vi "Fire Private Event.vi"(7 "AdHoc Cmd (\"\")":string, 8 "error in (no error)":errorcluster, 9 "vData":variant, 10 "PrivAsync":T1, 11 "Main in":refnum<class "Main.lvclass">) -> (0 "error out":errorcluster, 3 "Main out":refnum<class "Main.lvclass">)   [LabVIEW 2019, in "Main.lvclass"]
doc: "Developed by Kevin Thompson\nkevin@thompsonengineering.net\n\nCopyright 2018\nThompson Engineering, LLC"
uses:
  Main.lvclass
  DataTypes/PrivateAsynEv_Main--enum.ctl
  Common/DataTypes/TD Async CmdMsg EventData--cluster.ctl
  Main.lvclass/Main.ctl
  Accessors/Get ObjData.vi
  Config/Config.lvclass
  DAQ_Engine/DAQ_Engine.lvclass
  Log_Engine/Log_Engine.lvclass
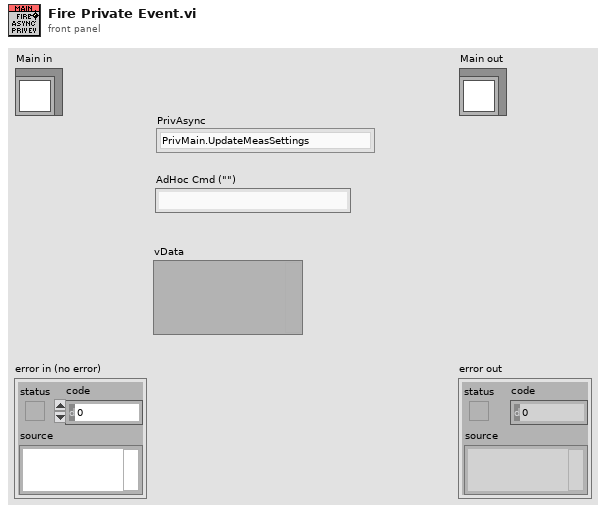
[diagram p1: front panel]
types:
  T1 = typedef "Main.lvclass/PrivateAsynEv_Main--enum.ctl" = enum16{"PrivMain.UpdateMeasSettings", "PrivMain.UpdateAcqMode", "PrivMain.UpdateDAQState", "PrivMain.UpdateLogState", "PrivMain.UpdateTDMSState", "PrivMain.UpdateProcessingState", "PrivMain.Stop&Terminate", "PrivMain.CurrInverterUpdated", "PrivMain.UpdateStoreUseESRBaseline", "PrivMain.SetUnsetAlarm&ESRBLine", "PrivMain.ResetAveraging"}
  T2 = typedef "TD Async CmdMsg EventData--cluster.ctl" = cluster{"Time Stamp":timestamp, "CmdMsg":string, "vData":variant}
  T3 = typedef "Main.lvclass/ObjData--cluster.ctl" = cluster{"Settings":T4, "Public Events":T7, "Dependency":T8, "ReadData-placeholder":T9, "VISA-placeholder":refnum<visa-resource-name>, "InverterWaveformsQ":T10, "Application.TerminateProcess Event":refnum<user-event>, "RawDaqDataQ":T11, "MeasSettings":T12, "InverterDataAcqMode":T13, "DAQState Data":T14, "Private Events":T16, "InvWfmsQ-DT":T10, "DPAuxDataQ":T17, "ProcessingState":T18, "InverterInfo":T19, "CurrInverters":T20[], "InverterLUT Dict":T24, "ESR Chart Ref":refnum<vi>[], "StoreESR BLine Ref":refnum<vi>, "UseSavedESR BLine Ref":refnum<vi>}
  T4 = typedef "Main.lvclass/Settings--cluster.ctl" = cluster{"Simulation":bool, "Signal scaling":T5[], "ESR scaling":T6[], "num readings to average":i32[], "ESR alarm threshhold (%)":i32[], "UseDummyVrms":bool, "Dummy Vrms":dbl, "Inverter Database File":path, "default Inverter (name)":string[]}
  T5 = typedef "Main.lvclass/Gain control.ctl" = cluster{"Iin ripple gain":dbl, "Iout ripple gain":dbl, "Iout 60Hz gain ":dbl, "Vout 60Hz gain ":dbl, "Iin ripple offest":dbl, "Iout ripple offset":dbl, "Iout 60Hz offset":dbl, "Vout 60Hz offset":dbl}
  T6 = typedef "Main.lvclass/ESR scaling--cluster.ctl" = cluster{"Gain":dbl, "Offset":dbl}
  T7 = typedef "Main.lvclass/Public Events--cluster.ctl" = cluster{"Main.AsyncCmd Event":refnum<user-event>, "Main.AsyncMsg Event":refnum<user-event>, "stop process":refnum<user-event>, "UpdateControlValue Ev":refnum<user-event>, "ProcessingStateChg Ev":refnum<user-event>}
  T8 = typedef "Main.lvclass/Dependency--cluster.ctl" = cluster{"Config":refnum<class "Config.lvclass">, "DAQ":refnum<class "DAQ_Engine.lvclass">, "Log_Engine":refnum<class "Log_Engine.lvclass">}
  T9 = typedef "Main.lvclass/Read Data--cluster.ctl" = cluster{"Data":dbl}
  T10 = typedef "InverterWaveforms--QRef.ctl" = refnum<queue>
  T11 = typedef "RawDAQDataQRef--cluster.ctl" = refnum<queue>
  T12 = typedef "Measurement Config--cluster.ctl" = cluster{"Data Rate 9775":dbl, "Data Rate 9215":dbl, "Samples RMS 9215":u32, "Samples RMS 9775":u32}
  T13 = typedef "Acquisition Mode--cluster.ctl" = enum16{"3phase", "Single"}
  T14 = typedef "DAQ_Engine.lvclass/DAQStateEvData--cluster.ctl" = cluster{"DAQState":T15, "vData":variant}
  T15 = typedef "DAQState--enum.ctl" = enum16{"Unknown", "Stopped", "Running", "Error"}
  T16 = typedef "Main.lvclass/Private Events--cluster.ctl" = cluster{"PrivateAsync Ev":refnum<user-event>}
  T17 = typedef "DataProcAuxDat--Qref.ctl" = refnum<queue>
  T18 = typedef "Main.lvclass/ProcessingState--enum.ctl" = enum16{"Idle", "Starting", "Running", "Done", "Error"}
  T19 = typedef "InverterInfo--cluster.ctl" = cluster{"Inverter ID":string}
  T20 = typedef "Inverter database record v2--cluster.ctl" = cluster{"name":string, "last updated":timestamp, "type":string, "inverter Info":T21, "gain range":T22, "offset range":T23, "gain actual":dbl, "offset actual":dbl, "power level":dbl, "minimum current":dbl, "resistance single phase":dbl, "resistance 3 phase":dbl, "set flag":u16}
  T21 = typedef "inverter info v2--cluster.ctl" = cluster{"manufacturer":string, "model":string, "product":string, "serial":string, "power class":string, "year manf":string}
  T22 = typedef "inverter gain range--cluster.ctl" = cluster{"gain max":dbl, "gain min":dbl, "gain increment":dbl}
  T23 = typedef "inverter offset range--cluster.ctl" = cluster{"offset max":dbl, "offset min":dbl, "offset increment":dbl}
  T24 = typedef "TD Dynamic CVT DVR--ref.ctl" = refnum<data-value>
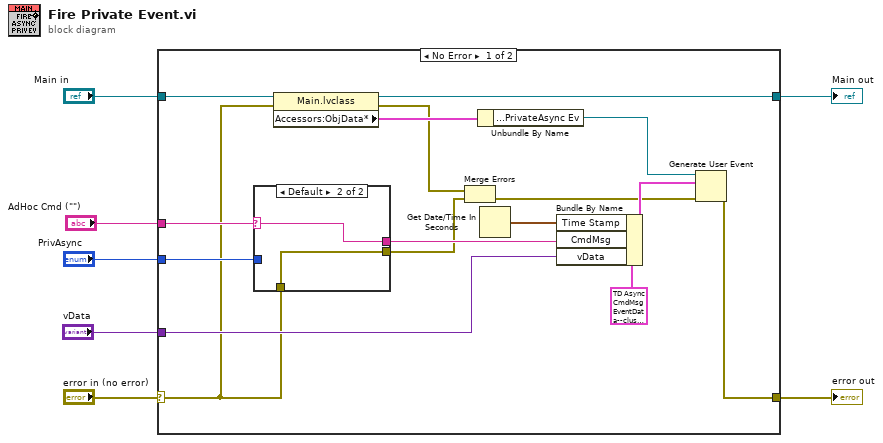
[diagram p0: block diagram]
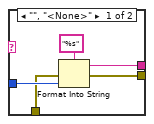
[diagram p2: hidden frame]
diagram:
  n1 = case shown="No Error" "error in (no error)" {
    selector: "error in (no error)" -> [w9 w32]
    tunnel: [w23 w32] -> w6
    tunnel: [w13 w31] -> w4
    tunnel: "Main in" -> [w14 w31]
    tunnel: "PrivAsync" -> [w17 _]
    tunnel: "vData" -> [w18 _]
    tunnel: "AdHoc Cmd (\"\")" -> [w16 _]
    frame No Error {
      n2 = case shown="Default" w16 {
        selector: w16 -> [_ w29]
        tunnel: w17 -> [w27 _]
        tunnel: [w26 w29] -> w19
        tunnel: w9 -> [w25 w30]
        tunnel: [w24 w30] -> w12
        frame "", "<None>" {
          n3 = Format Into String(format string="%s", error in=w25, w27) -> (resulting string=w26:string, error out=w24:errorcluster)  [unwired: 1 in]
        }
        frame Default {
        }
      }
      n4 = property class="Main.lvclass"(reference=w14, error in=w9) -> (reference out=w13:refnum<class "Main.lvclass">, error out=w10:errorcluster, "Accessors:ObjData*"=w15:T3)
      n5 = Merge Errors(w10, w12) -> (w11:errorcluster)
      n6 = Unbundle By Name(w15) -> ("Private Events.PrivateAsync Ev"=w8:refnum<user-event>)
      n7 = Get Date/Time In Seconds() -> (seconds since 1Jan1904=w20:timestamp)
      n8 = Bundle By Name(cluster=T2 {"Time Stamp"=timestamp(0 s since 1904-01-01), "CmdMsg"="", "vData"=variant} ("Async EvData"), "Time Stamp"=w20, "CmdMsg"=w19, "vData"=w18) -> (w22:T2)
      n9 = Generate User Event(user event=w8, event data cluster=w22, error in=w11) -> (error out=w23:errorcluster)  [unwired: 1 in, 1 out]
    }
    frame Error {
    }
  }
  "error out" <- w6
  "Main out" <- w4
